vi "Pins Names Write.vi"(4 "error in (no error)":errorcluster, 5 "Value":string[](array[string]), 6 "Container State":T2, 7 "Display State In":T1) -> (0 "error out":errorcluster, 3 "Display State Out":T1)   [LabVIEW 2021, in "roboRIO 10 Bank.xctl"]
uses:
  <vilib>/myRIO/Common/Instrument Driver Framework/Utilities/xctls/roboRIO 10 Bank/roboRIO 10 Bank.xctl
  <vilib>/_xctls/Container State.ctl
  <vilib>/myRIO/Common/Instrument Driver Framework/Utilities/xctls/roboRIO 10 Bank/State.ctl
  <vilib>/myRIO/Common/Instrument Driver Framework/Utilities/xctls/utilities/vis/myRIOXC Error Strings Global.vi
  <vilib>/_xctls/XControlSupport.lvlib
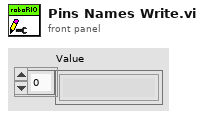
[diagram p1: front panel]
types:
  T1 = typedef "roboRIO 10 Bank.xctl/State.ctl" = cluster{"Pin Disabled?":enum8{"Enabled", "Disabled", "Disabled and Grayed Out"}[], "Pin Name":string[], "Pin ID":string[], "Connector Name":string, "Row Name 1":string, "Row Name 2":string}
  T2 = typedef "XControlSupport.lvlib/Container State.ctl" = cluster{"Indicator?":bool, "Run Mode?":bool, " Refnum":refnum<vi>}
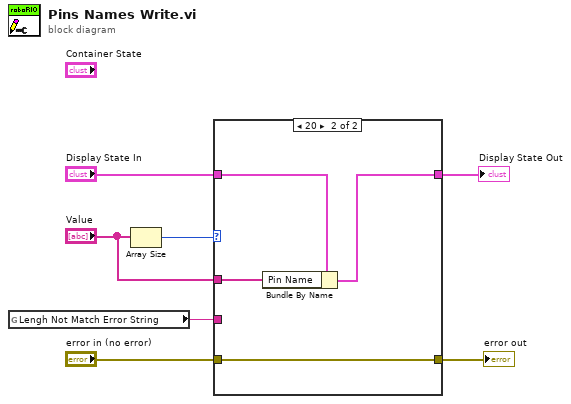
[diagram p0: block diagram]
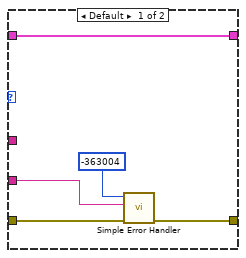
[diagram p2: hidden frame]
diagram:
  n1 = global read "myRIOXC Error Strings Global.vi" "Lengh Not Match Error String"() -> (w3:string)
  n2 = Array Size(array="Value") -> (size(s)=w7:i32)
  n3 = case shown="20" w7 {
    tunnel: "Value" -> [_ w13]
    tunnel: "Display State In" -> [w12 w15]
    tunnel: [w12 w14] -> w2
    tunnel: "error in (no error)" -> [w11 w16]
    tunnel: [w9 w16] -> w1
    tunnel: w3 -> [w8 _]
    frame Default {
      n4 = call <vilib>:"Simple Error Handler.vi"("error code (no error:0)"=-363004, "error source (\" \")"=w8, "error in (no error)"=w11) -> ("error out"=w9:errorcluster)  [unwired: 2 in, 4 out]
    }
    frame 20 {
      n5 = Bundle By Name(cluster=w15, "Pin Name"=w13) -> (w14:T1)
    }
  }
  "error out" <- w1
  "Display State Out" <- w2
